vi "TIC Read Gauge Pressure or Volts.vi"(0 "VISA Session In":refnum<visa-resource-name>, 5 "Gauge Number (1)":T1, 11 "error in (no error)":errorcluster) -> (4 "VISA Session (Dup)":refnum<visa-resource-name>, 6 "Gauge Number (Dup)":T1, 8 "Reading":dbl format="%.3e", 10 "Units":T2=enum."Volts", 15 "error out":errorcluster)   [LabVIEW 2018]
doc: "Returns the current pressure / voltage reading from the selected gauge."
uses:
  Turbo Instrument Controller.llb/Type Def - Gauge Num Selection.ctl
  Turbo Instrument Controller.llb/Type Def - Units.ctl
panel:
  out "mbar":dbl
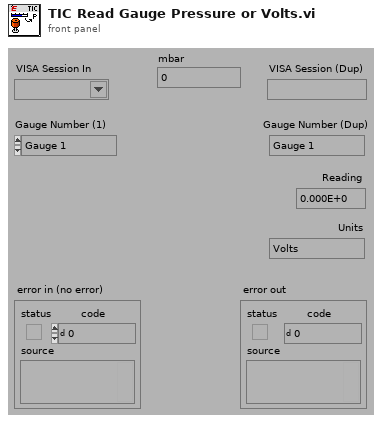
[diagram p1: front panel]
types:
  T1 = typedef "Type Def - Gauge Num Selection.ctl" = enum16{"Gauge 1", "Gauge 2", "Gauge 3", "Gauge 4", "Gauge 5", "Gauge 6"}
  T2 = typedef "Type Def - Units.ctl" = enum16{"Unknown", "Volts", "Pascals", "Percent"}
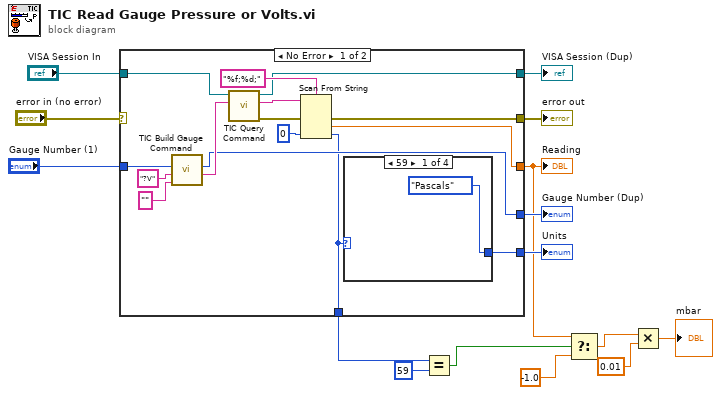
[diagram p0: block diagram]
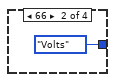
[diagram p2: hidden frame]
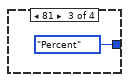
[diagram p3: hidden frame]
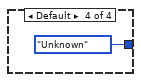
[diagram p4: hidden frame]
diagram:
  n1 = case shown="No Error" "error in (no error)" {
    selector: "error in (no error)" -> [_ w36]
    tunnel: "VISA Session In" -> [w25 w37]
    tunnel: [w24 w37] -> w14
    tunnel: "Gauge Number (1)" -> [w20 w35]
    tunnel: [w30 _] -> w8
    tunnel: [w29 w36] -> w12
    tunnel: [w27 _] -> w11
    tunnel: [w18 w35] -> w9
    tunnel: [w16 _] -> w5
    frame No Error {
      n2 = call "TIC Build Gauge Command.vi"("Command Suffix"="", "Command Prefix"="?V", "Gauge Number (1)"=w20) -> ("Command String"=w19:string, "Gauge Number (Dup)"=w18:T1)  [unwired: 7 in]
      n3 = call "TIC Query Command.vi"("Command String"=w19, "VISA Resource Name"=w25) -> ("error out"=w22:errorcluster, "Truncated Respose"=w23:string, "VISA session (Dup)"=w24:refnum<visa-resource-name>)  [unwired: 7 in]
      n4 = Scan From String(format string="%f;%d;", input string=w23, error in=w22, default 2=0) -> (error out=w29:errorcluster, output 1=w30:dbl, output 2=w16:i32)  [unwired: 2 in, 2 out]
      n5 = case shown="59" w16 {
        tunnel: [Type_Def_-_Units."Pascals" ("Units") Type_Def_-_Units."Volts" ("Units") Type_Def_-_Units."Percent" ("Units") Type_Def_-_Units."Unknown" ("Units")] -> w27
        frame 59 {
        }
        frame 66 {
        }
        frame 81 {
        }
        frame Default {
        }
      }
    }
    frame Error {
    }
  }
  "VISA Session (Dup)" <- w14
  "error out" <- w12
  "Reading" <- w8
  "Units" <- w11
  "Gauge Number (Dup)" <- w9
  n6 = Equal?(x=w5, y=59) -> (x = y?=w6:bool)
  n7 = Select(t=w8, s=w6, f=-1.0) -> (s? t:f=w3:dbl)
  n8 = Multiply(x=w3, y=0.01) -> (x*y=→"mbar":dbl)
